vi "Sonic Shifter Toggle.vi"   [LabVIEW 2013]
uses:
  Pneumatic Practice/State Machine Enum.ctl
  <vilib>/Rock Robotics/SystemInterfaces/Typedef/FPGA_TypedefSolenoidModule.ctl
  <vilib>/Rock Robotics/WPI/Solenoid/WPI_SolenoidChannel.ctl
  <vilib>/Rock Robotics/WPI/Solenoid/WPI_SolenoidValue.ctl
  <vilib>/Rock Robotics/WPI/Solenoid/WPI_SolenoidOpenSingle.vi
  Robot Global Data.vi
  <vilib>/Rock Robotics/WPI/Solenoid/WPI_SolenoidSetEnum.vi
types:
  T1 = typedef "State Machine Enum.ctl" = enum16{"Init", "Actuate", "Retract"}
  T2 = typedef "WPI_SolenoidChannel.ctl" = enum8{"Solenoid 1", "Solenoid 2", "Solenoid 3", "Solenoid 4", "Solenoid 5", "Solenoid 6", "Solenoid 7", "Solenoid 8", "Invalid"}
  T3 = typedef "FPGA_TypedefSolenoidModule.ctl" = enum16{"Solenoid Module 1", "Solenoid Module 2"}
  T4 = typedef "WPI_SolenoidValue.ctl" = enum16{"Off", "On", "Forward", "Reverse"}
  T5 = typedef "WPI_SolenoidDevRef.ctl" = cluster{"DevStatus":errorcluster, "Solenoid Module":T3, "Forward Solenoid Channel":T2, "Reverse Solenoid Channel":T2}
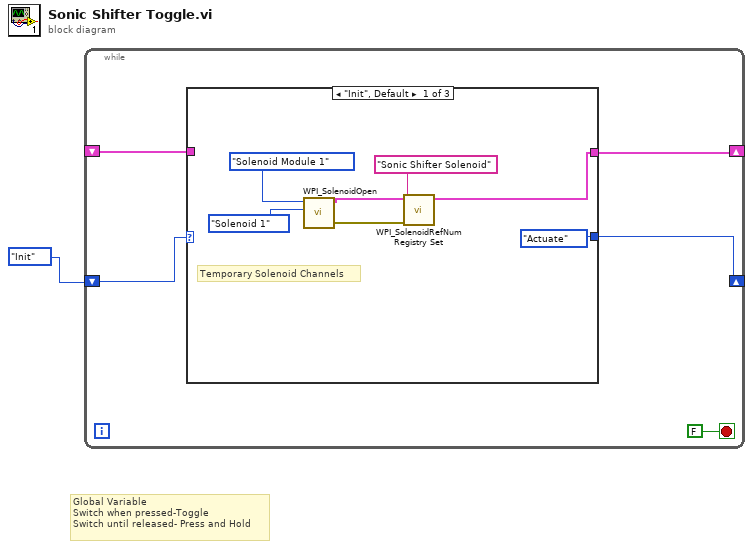
[diagram p0: block diagram]
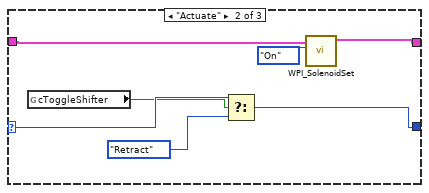
[diagram p2: hidden frame]
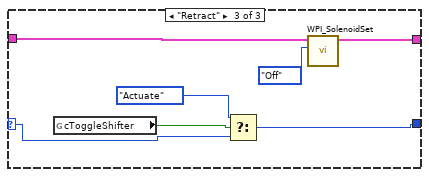
[diagram p3: hidden frame]
diagram:
  # "Global Variable\nSwitch when pressed-Toggle\nSwitch until released- Press and Hold"
  n1 = while {
    shift-right: [w5] -> _
    shift-left: State_Machine_Enum."Init" -> [w6]
    shift-right: [w4] -> _
    shift-left: _ -> [w3]
    stop <- FALSE stop-if-true
    n2 = case shown="\"Init\", Default" w6 {
      selector: w6 -> [_ w15 w21]
      tunnel: [State_Machine_Enum."Actuate" w17 w22] -> w5
      tunnel: [w9 w20 w24] -> w4
      tunnel: w3 -> [_ w19 w25]
      frame "Init", Default {
        # "Temporary Solenoid Channels"
        n3 = call-poly <vilib>:"WPI_SolenoidOpen.vi"("Solenoid Channel"=WPI_SolenoidChannel."Solenoid 1", "Solenoid Module (Module 1)"=FPGA_TypedefSolenoidModule."Solenoid Module 1") -> ("error out"=w7:errorcluster, "SolenoidDevRef"=w10:T5)  [unwired: 8 in]
        n4 = call <vilib>:"WPI_SolenoidRefNum Registry Set.vi"("error in (no error)"=w7, "refnum name"="Sonic Shifter Solenoid", "SolenoidDevRef"=w10) -> ("SolenoidDevRef"=w9:T5)  [unwired: 7 in, 1 out]
      }
      frame "Actuate" {
        n5 = global read "Robot Global Data.vi" "cToggleShifter"() -> (w14:bool)
        n6 = Select(t=w15, s=w14, f=State_Machine_Enum."Retract") -> (s? t:f=w17:T1)
        n7 = call-poly <vilib>:"WPI_SolenoidSet.vi"("Value"=WPI_SolenoidValue."On", "SolenoidDevRef"=w19) -> ("SolenoidDevRef"=w20:T5)  [unwired: 8 in, 1 out]
      }
      frame "Retract" {
        n8 = global read "Robot Global Data.vi" "cToggleShifter"() -> (w27:bool)
        n9 = Select(t=State_Machine_Enum."Actuate", s=w27, f=w21) -> (s? t:f=w22:T1)
        n10 = call-poly <vilib>:"WPI_SolenoidSet.vi"("Value"=WPI_SolenoidValue."Off", "SolenoidDevRef"=w25) -> ("SolenoidDevRef"=w24:T5)  [unwired: 8 in, 1 out]
      }
    }
  }
